vi "Write to File.vi"(8 "error in":errorcluster, 10 "File Actor In":refnum<class "File Actor.lvclass">, 11 "Exe Write Main in":refnum<class "Exe Write Main.lvclass">) -> (0 "error out":errorcluster, 2 "File Actor Out":refnum<class "File Actor.lvclass">)   [LabVIEW 2018, in "Controller.lvlib" / "Exe Write Main.lvclass"]
doc: "In this command, we pole the MAP DVR which contains all of the data that is to be written to file...."
uses:
  Exe Write Main.lvclass
  File Actor/File Actor.lvclass
  C:/Users/Labview/Documents/exscalabar_server/SuperActor/SuperActor.lvclass
  File Actor/File Actor.lvclass/File Actor.ctl
  SuperActor/SuperActor.lvclass/SuperActor.ctl
  Exe Write Main.lvclass/Exe Write Main.ctl
  File Actor/Read Save DVR.vi
  File Actor/Read File DVR.vi
  SuperActor/Read Log Session.vi
  <userlib>/_Session Fwk/Session - Root.lvclass
  reusable/Session APIs/Session Log/System Log.lvclass
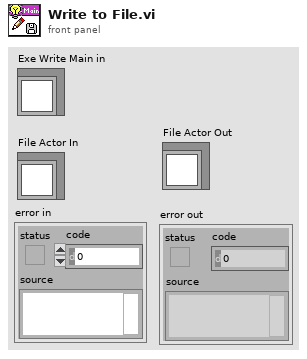
[diagram p1: front panel]
types:
  T1 = typedef "Session - Root.lvclass/Session Handle.ctl" = refnum<data-value>
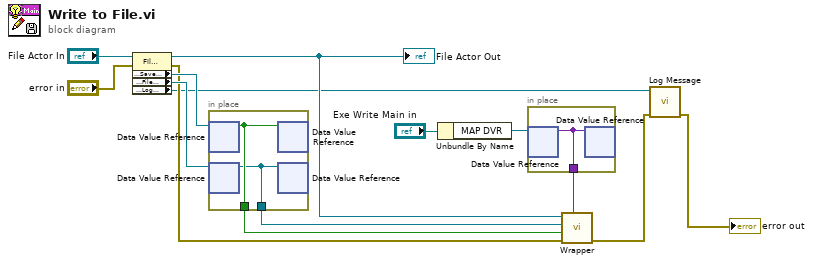
[diagram p0: block diagram]
diagram:
  n1 = property class="File Actor"(reference="File Actor In", error in="error in") -> (reference out=w4:refnum<class "File Actor.lvclass">, error out=w8:errorcluster, "Accessors:Save DVR"=w13:refnum<data-value>, "Accessors:File DVR"=w11:refnum<data-value>, "Accessors:Log Session"=w3:T1)
  "File Actor Out" <- w4
  n2 = in-place {
    in-place-border: [w16] -> w12
    in-place-border: [w15] -> w10
    n3 = in-place-dvr #1(w13) -> (w16:bool)  [unwired: 1 out]
    n4 = in-place-dvr #2(w11) -> (w15:refnum<file>)  [unwired: 1 out]
    n5 = in-place-dvr #1(w16) -> ()  [unwired: 2 out]
    n6 = in-place-dvr #2(w15) -> ()  [unwired: 2 out]
  }
  n7 = Unbundle By Name("Exe Write Main in") -> ("MAP DVR"=w6:refnum<data-value>)
  n8 = in-place {
    in-place-border: [w17] -> w5
    n9 = in-place-dvr #3(w6) -> (w17:variant)  [unwired: 1 out]
    n10 = in-place-dvr #3(w17) -> ()  [unwired: 2 out]
  }
  n11 = call "Wrapper.vi"("Data Map"=w5, "error in"=w8, "Save?"=w12, "File Ref"=w10, "File Actor in"=w4) -> ("error out"=w2:errorcluster)  [unwired: 6 in]
  n12 = call "Log Message.vi"("error in"=w2, "session in"=w3) -> ("error out"=→"error out":errorcluster)  [unwired: 8 in, 1 out]
